vi "_WCA_CLNA_Sweep.vi"(8 "CLNAsweep":T3={"VDmin"=1.0, "VDmax"=2.0, "VDstep"=0.1, "IDmin"=8.0, "IDmax"=20.0, "IDstep"=1.0, "wait (mS)"=500.0, "P.M.aveg"=10, "HOT/COLD "=0, "SIS hotV "=8.0, "SIS coldV"=5.0, "file_name"="", "frq(GHz)"=8.0} {"HOT/COLD" items=["Liq Ni Motor", "SISBias"]}, 10 "Control":T2={"GPIB_ATT"="28", "6501Dev#"=1, "GPIB_SP"="18", "GPIB_PM"="13", "GPIB_DSA"="11", "GPIB_DMM (TPD)"="23", "GPIB_MPI"="2", "mortor設定"=[{"Axis"=0, "ID"=0, "HIspeed"=200.0, "LOspeed"=100.0, "ACCEL(ms)"=100.0, "Sratio"=50.0, "フリーラン\n"=TRUE, "文字列"="DSB HOT/COLD"}, {"Axis"=1, "ID"=0, "HIspeed"=4.0, "LOspeed"=4.0, "ACCEL(ms)"=100.0, "Sratio"=50.0, "フリーラン\n"=TRUE, "文字列"="SubMM Att"}], "DATAパス"=path "Z:/band10/Labview_ALMA/MIX95/test", "DBパス "=path "Z:/band10/Labview_ALMA/MIX95/test", "comment"="P1_Tmin", "ColdCarts"="003601", "Th"=295.0, "Tc"=77.0, "Set_SIS_volt"=2.1, "Offset"=0.0, "control"=0, "FreqLO"=800.0, "Set_Mag_Cur"=800.0, "MPI offset(mm)"=22.99, "HOT/COLD"=0} {"HOT/COLD" items=["DSB", "SBR", "GainComp"]; "control" items=["CLOSE LOOP", "OPEN LOOP", "Not Control"]}, 11 "Bias_LO_equip":T1={"Node address"=19, "CAN Interface"="CAN0", "Cartridge band"=10, "Slave Node in"={"Address"=0, "Serial Number"=[]}, "ObjHandle out"=0, "POL"=1, "sb"=1, "GPIB_SM (SIS S,V)"="24", "GPIB_DMM (SIS I)"="22", "GPIB_SM (MAG I) "="25", "GPIB_SG(LO)"="19", "GPIB_PW (PAMP) "="6", "GPIB_TMP1(8ch)"="12", "GPIB_TMP2(2ch)  "="13", "WCA_avg"=10, "Rsen"=10.0, "BiasModule"=1, "LOModule "=1, "WCA_LO_FREQ_SET"={"YTO Low freq. [GHz]"=14.42, "YTO High freq. [GHz]"=17.7, "Kvco"=1, "Lock Pol."=0, "SET LO FREQ"=72.5, "Multiplier"=6.0, "YTO (HEX)"=0, "YTO coarse( FREQ)"=25.0, "NULL PLL INTEGRATOR"=FALSE}, "Res for"=0} {"Res for" items=["none", "series res", "parallel res"]; "WCA_LO_FREQ_SET"."YTO coarse( FREQ)" min=25 max=150 step=0.0001 format="%.3f"; "WCA_LO_FREQ_SET"."Multiplier" min=3 max=6 step=3; "WCA_LO_FREQ_SET"."SET LO FREQ" min=25 max=150 step=0.0001 format="%.3f"; "WCA_LO_FREQ_SET"."Lock Pol." items=["Lower", "Upper"]; "WCA_LO_FREQ_SET"."Kvco" items=["7.5MHz/V", "15MHz/V"]; "WCA_LO_FREQ_SET"."YTO High freq. [GHz]" format="%.3f"; "WCA_LO_FREQ_SET"."YTO Low freq. [GHz]" format="%.3f"; "LOModule" items=["Manual", "B10Lab LO", "WCA LO"]; "BiasModule" items=["B10Lab Bias", "WCA BiasModule"]; "Slave Node in"."Serial Number" format="%.0x"; "Slave Node in"."Address" format="%.0x"; "Cartridge band" max=10 step=1; "Node address" format="%.0x"}) -> ()   [LabVIEW 2017]
uses:
  __sub_vi/WCA_NAOJ_sub_vi/WCA_Global.vi
  Instance           2 23Saved   _WCA_CLNA_Sweep .vi
  Instance           4 23Saved   _WCA_CLNA_Sweep .vi
  <vilib>/Utility/file.llb/Write To Spreadsheet File (DBL).vi
  <vilib>/express/express shared/transition.llb/Dynamic To Waveform Array.vi
  <vilib>/express/express arith-compare/Formula/Block/exnFormulaBlock how many pts in the wave.vi
  <vilib>/express/express shared/ex_Modify Signal Name.vi
  <vilib>/express/express shared/transition.llb/Waveform Array To Dynamic.vi
  Instance           3 23Saved   _WCA_CLNA_Sweep .vi
  <vilib>/express/express arith-compare/Formula/XNode/ExpressFormulaBlockNode.xnode
panel:
  in  "タブ制御器":enum32{"機器セッティング", "ページ 2", "ページ 3", "ページ 4"}(tab)
  out "Y_":dbl=-0.021313399999996818
  out "Phot":dbl=-36.0813292
  out "Pcold":dbl=-36.0600158
  out "Get VG":dbl=-3.6497344970703125
  out "Get ID":dbl=25.091552734375
  out "Get VD":dbl=2.003662109375
  out "Set ID":dbl=20.0
  out "Set VD":dbl=2.0
  out "error out":errorcluster={"status"=TRUE, "code"=-1074388991, "source"="NI-CAN Wait For State\n(ncWait.vi)"} caption="エラー出力"
  out "Link済み":bool=TRUE
  in  "CLNA_SET":T4 {"SET POL0 LNA1 STAGE3 DRAIN C" min=0 max=20 step=0.01 format="%.2f"; "SET POL0 LNA1 STAGE3 DRAIN V" min=0 max=3 step=0.01 format="%.2f"; "SET POL0 LNA1 STAGE2 DRAIN C" min=0 max=20 step=0.01 format="%.2f"; "SET POL0 LNA1 STAGE2 DRAIN V" min=0 max=3 step=0.01 format="%.2f"; "SET POL0 LNA1 STAGE1 DRAIN C" min=0 max=20 step=0.01 format="%.2f"; "SET POL0 LNA1 STAGE1 DRAIN V" min=0 max=3 step=0.01 format="%.2f"; "CLNA State" items=["Disabled", "Enabled"]}
  out "AllDATA":dbl[][](array[numeric])=[[1.0023040771484375, 1.002105712890625, 1.0022430419921875, 1.0023345947265625, 1.002197265625, 1.0023040771484375, 1.0023956298828125, 1.002227783203125, 1.0021514892578125, 1.0023956298828125, 1.0024871826171875, 1.0022430419921875, 1.0022125244140625, 1.102142333984375, 1.10211181640625, 1.1022491455078125, 1.10211181640625, 1.102294921875, 1.1024169921875, 1.1022796630859375, 1.1022491455078125, 1.1023712158203125, 1.1024017333984375, 1.1024017333984375, 1.1022796630859375, 1.102294921875, 1.2026519775390625, 1.2027435302734375, 1.20269775390625, 1.2028045654296875, 1.2025299072265625, 1.202789306640625, 1.2028656005859375, 1.2028961181640625, 1.2029266357421875, 1.2028656005859375, 1.2026519775390625, 1.2027740478515625, 1.2029266357421875, 1.302642822265625, 1.302703857421875, 1.3027191162109375, 1.302764892578125, 1.3028106689453125, 1.30279541015625, 1.3028106689453125, 1.302978515625, 1.3027496337890625, 1.302825927734375, 1.302642822265625, 1.30291748046875, 1.3028411865234375, 1.4028472900390625, 1.4030914306640625, 1.403167724609375, 1.4028472900390625, 1.4028778076171875, 1.4028778076171875, 1.402679443359375, 1.403076171875, 1.402679443359375, 1.40301513671875, 1.4030914306640625, 1.402984619140625, 1.4026641845703125, 1.503662109375, 1.5032196044921875, 1.50323486328125, 1.5030517578125, 1.5032958984375, 1.5032806396484375, 1.5030364990234375, 1.50335693359375, 1.5030975341796875, 1.5032501220703125, 1.5030517578125, 1.503204345703125, 1.5032196044921875, 1.60296630859375, 1.6030731201171875, 1.603363037109375, 1.6032562255859375, 1.603179931640625, 1.60296630859375, 1.60308837890625, 1.6032562255859375, 1.60308837890625, 1.60321044921875, 1.60321044921875, 1.603057861328125, 1.603118896484375, 1.7034912109375, 1.703216552734375, 1.7032470703125, 1.7033538818359375, 1.7030181884765625, 1.7031097412109375, 1.703460693359375, 1.7033538818359375, 1.70318603515625, 1.7034149169921875, 1.7034759521484375, 1.70306396484375, 1.70343017578125, 1.803375244140625, 1.8035430908203125, 1.8034210205078125, 1.8034515380859375, 1.80340576171875, 1.8035736083984375, 1.8033599853515625, 1.803466796875, 1.8035125732421875, 1.8033599853515625, 1.8035888671875, 1.8033905029296875, 1.8037109375, 1.903350830078125, 1.903472900390625, 1.9034576416015625], [8.008880615234375, 9.035491943359375, 9.97100830078125, 11.0247802734375, 12.0404052734375, 13.050689697265625, 14.05731201171875, 15.0653076171875, 16.02996826171875, 17.058563232421875, 18.0487060546875, 19.04052734375, 20.05828857421875, 8.039398193359375, 8.996124267578125, 10.06439208984375, 11.038818359375, 12.03704833984375, 13.03802490234375, 14.0863037109375, 15.06439208984375, 16.061859130859375, 17.065887451171875, 18.072052001953125, 19.047698974609375, 20.0762939453125, 8.032989501953125, 9.056243896484375, 10.06011962890625, 11.0638427734375, 12.0782470703125, 13.007965087890625, 14.0386962890625, 15.06439208984375, 16.035308837890625, 17.039337158203125, 18.033905029296875, 19.078369140625, 20.070037841796875, 8.048248291015625, 9.024200439453125, 9.9859619140625, 11.053009033203125, 12.051239013671875, 13.049468994140625, 14.071807861328125, 15.03143310546875, 16.085052490234375, 17.037353515625, 18.03558349609375, 19.07135009765625, 20.034027099609375, 7.994232177734375, 9.02862548828125, 10.037841796875, 11.07452392578125, 12.032928466796875, 13.063507080078125, 14.0386962890625, 15.02197265625, 16.014404296875, 17.052001953125, 18.072662353515625, 19.047393798828125, 20.04119873046875, 5.80596923828125, 3.686065673828125, 5.312347412109375, 4.949188232421875, 16.232452392578125, 13.04046630859375, 14.048919677734375, 15.037078857421875, 16.081695556640625, 17.0587158203125, 18.0523681640625, 19.07867431640625, 20.0244140625, 13.279266357421875, 6.36016845703125, 4.31121826171875, 7.32452392578125, 6.24359130859375, 7.073822021484375, 18.690032958984375, 15.014190673828125, 16.087799072265625, 17.076568603515625, 18.069305419921875, 19.0643310546875, 20.07080078125, 8.0560302734375, 8.16162109375, 3.512115478515625, 5.3619384765625, 20.580902099609375, 20.821380615234375, 16.0015869140625, 4.630889892578125, 15.82916259765625, 17.030029296875, 18.027801513671875, 19.0692138671875, 20.095367431640625, 21.844635009765625, 21.697540283203125, 21.622772216796875, 21.66259765625, 21.610870361328125, 21.63330078125, 21.61102294921875, 21.68212890625, 21.672210693359375, 21.784210205078125, 21.6229248046875, 19.026336669921875, 20.05340576171875, 23.668670654296875, 23.538970947265625, 23.544464111328125], [0.7330169677734375, 0.8783721923828125, 1.0079498291015625, 1.1290283203125, 1.2441253662109375, 1.350372314453125, 1.4566192626953125, 1.5489501953125, 1.6483917236328125, 1.746734619140625, 1.853759765625, 1.9870452880859375, 2.1604461669921875, 0.525146484375, 0.680755615234375, 0.8156890869140625, 0.9432830810546875, 1.061859130859375, 1.179656982421875, 1.2897186279296875, 1.4064178466796875, 1.506317138671875, 1.6030120849609375, 1.69744873046875, 1.7970123291015625, 1.901336669921875, 0.2288360595703125, 0.406005859375, 0.5797576904296875, 0.7351226806640625, 0.872039794921875, 0.9920654296875, 1.1099395751953125, 1.22442626953125, 1.33905029296875, 1.4532470703125, 1.55426025390625, 1.6502532958984375, 1.7432403564453125, -0.0763092041015625, 0.1149749755859375, 0.2913055419921875, 0.4664764404296875, 0.630157470703125, 0.7830963134765625, 0.91229248046875, 1.037567138671875, 1.1466217041015625, 1.265960693359375, 1.378326416015625, 1.4917755126953125, 1.594451904296875, -0.3813323974609375, -0.1755523681640625, 0.013671875, 0.186920166015625, 0.349578857421875, 0.50616455078125, 0.6645050048828125, 0.818389892578125, 0.9545440673828125, 1.0711212158203125, 1.1864166259765625, 1.303497314453125, 1.4156951904296875, -1.2528839111328125, -1.786773681640625, -1.2420196533203125, -1.305328369140625, -1.882781982421875, 0.2266998291015625, 0.3792724609375, 0.535247802734375, 0.6952362060546875, 0.84088134765625, 0.9810943603515625, 1.1031036376953125, 1.21795654296875, -2.3688201904296875, -1.410064697265625, -2.0248565673828125, -1.0382232666015625, -1.1384124755859375, -1.006744384765625, -2.1786651611328125, 0.3073883056640625, 0.4534149169921875, 0.5962371826171875, 0.748260498046875, 0.8952178955078125, 1.03143310546875, -1.3086395263671875, -1.2085418701171875, -2.661956787109375, -2.0058746337890625, -2.78607177734375, -3.555145263671875, -1.39764404296875, -1.9747161865234375, -1.3009796142578125, 0.34893798828125, 0.4822540283203125, 0.62396240234375, 0.7726287841796875, -3.6534423828125, -3.6532135009765625, -3.653228759765625, -3.6531982421875, -3.6529541015625, -3.652801513671875, -3.6527252197265625, -3.652679443359375, -3.652496337890625, -3.6523590087890625, -3.652435302734375, 0.3907623291015625, 0.527252197265625, -3.65203857421875, -3.6520233154296875, -3.65191650390625], [-15.8019747, -14.345305, -13.3210423, -12.5917133, -12.0920286, -11.7980894, -11.6930614, -11.7846915, -12.0721581, -12.6224904, -13.7267507, -16.5712959, -21.5777376, -17.0933087, -15.2334231, -13.8489237, -12.8692605, -12.1592133, -11.639288, -11.2830662, -11.0867126, -11.0497694, -11.1765261, -11.5024369, -12.0712356, -13.1210202, -18.6468403, -16.1476854, -14.570121, -13.4081903, -12.4958806, -11.8057103, -11.2893617, -10.90672, -10.6370429, -10.4946825, -10.494992, -10.6523369, -10.9887522, -22.5221729, -18.125333, -15.4214337, -13.9034386, -12.8769868, -12.1038889, -11.4548295, -10.9493002, -10.5603601, -10.272209, -10.0697857, -9.98018936, -10.0091371, -27.7214104, -22.9626936, -18.0779783, -15.2169109, -13.537981, -12.4632357, -11.7336743, -11.1640832, -10.6783089, -10.3048974, -10.0043142, -9.78552749, -9.63525648, -29.9236072, -30.0847895, -30.3171631, -30.3069408, -30.5019806, -13.4081314, -12.1836691, -11.3858437, -10.8426287, -10.4020521, -10.0248496, -9.71805946, -9.50416462, -28.864449, -30.5298938, -29.3480611, -30.7227796, -30.9749093, -30.1810534, -30.4759237, -11.8363611, -11.0494144, -10.4770986, -10.0581157, -9.73425389, -9.45626546, -28.7626425, -29.4905465, -28.7472986, -30.4154173, -29.8859621, -31.9666589, -30.5494954, -30.5235955, -31.7679326, -10.9375712, -10.3127095, -9.84276742, -9.48202177, -34.5858391, -34.5288413, -34.3235417, -34.3295835, -34.5159358, -34.3741306, -34.4705043, -34.5540513, -34.4242323, -34.5184065, -27.8331629, -10.1602425, -9.68344682, -35.2753216, -35.3063507, -35.2783414], [-18.1174805, -16.6835391, -15.6987861, -14.9944898, -14.5063113, -14.2123343, -14.104885, -14.1915152, -14.4719556, -15.0076862, -16.0726006, -18.7799405, -23.2595732, -19.2586723, -17.5333956, -16.2048421, -15.2456024, -14.556834, -14.049878, -13.692676, -13.4852123, -13.4535138, -13.5758048, -13.8915443, -14.4403795, -15.4600873, -20.6351209, -18.3316269, -16.8141631, -15.7405915, -14.8552992, -14.1820555, -13.6803907, -13.296921, -13.0340352, -12.8908561, -12.8921382, -13.0431259, -13.3727695, -23.9303013, -20.0681201, -17.6391096, -16.1885809, -15.2049061, -14.4666364, -13.8254901, -13.3183269, -12.9474389, -12.6593856, -12.4648366, -12.3737855, -12.6038004, -27.8709028, -24.0548698, -19.9170932, -17.3075996, -15.8115317, -14.7876725, -14.079908, -13.527917, -13.0683468, -12.6767887, -12.3950819, -12.1703213, -12.0184709, -29.8978082, -29.5950189, -30.1216617, -30.2923534, -30.7282828, -15.6183781, -14.4711486, -13.7208693, -13.1918311, -12.762488, -12.4131872, -12.1016409, -11.8839305, -28.9212261, -29.0167155, -29.6828341, -31.0176264, -30.2920578, -30.9538346, -30.4441937, -14.1155557, -13.3635281, -12.8309223, -12.4244692, -12.1112123, -11.8309856, -28.8106043, -30.8510766, -29.2806575, -31.1178272, -31.2416511, -29.5672254, -29.902671, -30.8986962, -31.7747404, -13.220053, -12.6236218, -12.1768264, -11.8501035, -34.4679122, -34.4354168, -28.5827453, -34.491634, -34.4472451, -34.5085919, -34.4868301, -34.2848253, -34.4136795, -34.4331047, -13.1088166, -12.4595201, -12.0024162, -35.4359339, -35.4317712, -35.3773834], [2.3155057999999986, 2.338234100000001, 2.3777437999999993, 2.4027765, 2.4142826999999993, 2.4142449, 2.4118236, 2.4068237000000003, 2.3997975, 2.3851958, 2.345849900000001, 2.2086445999999995, 1.6818355999999994, 2.165363599999999, 2.299972499999999, 2.3559184, 2.3763419, 2.397620700000001, 2.410589999999999, 2.4096098, 2.3984997000000003, 2.403744399999999, 2.3992787, 2.3891074000000003, 2.369143900000001, 2.3390670999999994, 1.9882805999999995, 2.1839414999999995, 2.244042099999998, 2.3324012000000014, 2.3594185999999997, 2.376345200000001, 2.3910289999999996, 2.3902009999999994, 2.396992299999999, 2.396173600000001, 2.3971462, 2.390789, 2.3840173, 1.408128399999999, 1.9427871000000003, 2.2176759000000015, 2.285142300000002, 2.3279193000000014, 2.362747500000001, 2.370660599999999, 2.369026700000001, 2.3870787999999994, 2.3871766, 2.3950508999999993, 2.3935961399999997, 2.5946633000000006, 0.14949239999999975, 1.0921761999999973, 1.8391148999999984, 2.0906886999999994, 2.2735506999999995, 2.324436799999999, 2.346233699999999, 2.3638338, 2.390037900000001, 2.3718912999999997, 2.3907676999999996, 2.3847938099999997, 2.38321442, -0.02579899999999924, -0.48977059999999994, -0.19550139999999772, -0.014587399999999917, 0.22630219999999923, 2.210246699999999, 2.2874795, 2.3350256, 2.3492023999999994, 2.360435899999999, 2.3883376, 2.3835814400000004, 2.3797658800000008, 0.056777099999997915, -1.5131782999999999, 0.334773000000002, 0.29484680000000196, -0.6828515000000017, 0.7727812000000007, -0.03172999999999959, 2.2791946000000003, 2.3141137, 2.3538236999999995, 2.3663535000000007, 2.3769584100000003, 2.374720140000001, 0.04796180000000305, 1.3605300999999983, 0.5333588999999996, 0.7024098999999993, 1.3556889999999981, -2.399433499999997, -0.6468243999999999, 0.37510070000000084, 0.006807799999997144, 2.2824817999999993, 2.3109123, 2.33405898, 2.36808173, -0.1179269000000005, -0.09342450000000468, -5.740796400000001, 0.16205049999999943, -0.06869069999999766, 0.13446129999999812, 0.01632579999999706, -0.2692259999999962, -0.010552799999999252, -0.08530179999999632, -14.7243463, 2.2992776, 2.3189693800000004, 0.16061230000000393, 0.12542049999999705, 0.09904199999999719]]
  out "GETID2d":dbl[][](array[numeric])=[[8.008880615234375, 9.035491943359375, 9.97100830078125, 11.0247802734375, 12.0404052734375, 13.050689697265625, 14.05731201171875, 15.0653076171875, 16.02996826171875, 17.058563232421875, 18.0487060546875, 19.04052734375, 20.05828857421875], [8.039398193359375, 8.996124267578125, 10.06439208984375, 11.038818359375, 12.03704833984375, 13.03802490234375, 14.0863037109375, 15.06439208984375, 16.061859130859375, 17.065887451171875, 18.072052001953125, 19.047698974609375, 20.0762939453125], [8.032989501953125, 9.056243896484375, 10.06011962890625, 11.0638427734375, 12.0782470703125, 13.007965087890625, 14.0386962890625, 15.06439208984375, 16.035308837890625, 17.039337158203125, 18.033905029296875, 19.078369140625, 20.070037841796875], [8.048248291015625, 9.024200439453125, 9.9859619140625, 11.053009033203125, 12.051239013671875, 13.049468994140625, 14.071807861328125, 15.03143310546875, 16.085052490234375, 17.037353515625, 18.03558349609375, 19.07135009765625, 20.034027099609375], [7.994232177734375, 9.02862548828125, 10.037841796875, 11.07452392578125, 12.032928466796875, 13.063507080078125, 14.0386962890625, 15.02197265625, 16.014404296875, 17.052001953125, 18.072662353515625, 19.047393798828125, 20.04119873046875], [5.80596923828125, 3.686065673828125, 5.312347412109375, 4.949188232421875, 16.232452392578125, 13.04046630859375, 14.048919677734375, 15.037078857421875, 16.081695556640625, 17.0587158203125, 18.0523681640625, 19.07867431640625, 20.0244140625], [13.279266357421875, 6.36016845703125, 4.31121826171875, 7.32452392578125, 6.24359130859375, 7.073822021484375, 18.690032958984375, 15.014190673828125, 16.087799072265625, 17.076568603515625, 18.069305419921875, 19.0643310546875, 20.07080078125], [8.0560302734375, 8.16162109375, 3.512115478515625, 5.3619384765625, 20.580902099609375, 20.821380615234375, 16.0015869140625, 4.630889892578125, 15.82916259765625, 17.030029296875, 18.027801513671875, 19.0692138671875, 20.095367431640625], [21.844635009765625, 21.697540283203125, 21.622772216796875, 21.66259765625, 21.610870361328125, 21.63330078125, 21.61102294921875, 21.68212890625, 21.672210693359375, 21.784210205078125, 21.6229248046875, 19.026336669921875, 20.05340576171875], [23.668670654296875, 23.538970947265625, 23.544464111328125, 23.495635986328125, 23.45367431640625, 23.48358154296875, 23.45367431640625, 23.459625244140625, 23.370819091796875, 23.431549072265625, 23.40972900390625, 23.4197998046875, 23.384552001953125], [25.102386474609375, 25.07843017578125, 25.081787109375, 25.060577392578125, 25.09002685546875, 25.065460205078125, 25.092620849609375, 25.110015869140625, 25.070648193359375, 25.105438232421875, 25.09002685546875, 25.069732666015625, 25.091552734375]]
  out "GetVD 2D":dbl[][](array[numeric])=[[1.0023040771484375, 1.002105712890625, 1.0022430419921875, 1.0023345947265625, 1.002197265625, 1.0023040771484375, 1.0023956298828125, 1.002227783203125, 1.0021514892578125, 1.0023956298828125, 1.0024871826171875, 1.0022430419921875, 1.0022125244140625], [1.102142333984375, 1.10211181640625, 1.1022491455078125, 1.10211181640625, 1.102294921875, 1.1024169921875, 1.1022796630859375, 1.1022491455078125, 1.1023712158203125, 1.1024017333984375, 1.1024017333984375, 1.1022796630859375, 1.102294921875], [1.2026519775390625, 1.2027435302734375, 1.20269775390625, 1.2028045654296875, 1.2025299072265625, 1.202789306640625, 1.2028656005859375, 1.2028961181640625, 1.2029266357421875, 1.2028656005859375, 1.2026519775390625, 1.2027740478515625, 1.2029266357421875], [1.302642822265625, 1.302703857421875, 1.3027191162109375, 1.302764892578125, 1.3028106689453125, 1.30279541015625, 1.3028106689453125, 1.302978515625, 1.3027496337890625, 1.302825927734375, 1.302642822265625, 1.30291748046875, 1.3028411865234375], [1.4028472900390625, 1.4030914306640625, 1.403167724609375, 1.4028472900390625, 1.4028778076171875, 1.4028778076171875, 1.402679443359375, 1.403076171875, 1.402679443359375, 1.40301513671875, 1.4030914306640625, 1.402984619140625, 1.4026641845703125], [1.503662109375, 1.5032196044921875, 1.50323486328125, 1.5030517578125, 1.5032958984375, 1.5032806396484375, 1.5030364990234375, 1.50335693359375, 1.5030975341796875, 1.5032501220703125, 1.5030517578125, 1.503204345703125, 1.5032196044921875], [1.60296630859375, 1.6030731201171875, 1.603363037109375, 1.6032562255859375, 1.603179931640625, 1.60296630859375, 1.60308837890625, 1.6032562255859375, 1.60308837890625, 1.60321044921875, 1.60321044921875, 1.603057861328125, 1.603118896484375], [1.7034912109375, 1.703216552734375, 1.7032470703125, 1.7033538818359375, 1.7030181884765625, 1.7031097412109375, 1.703460693359375, 1.7033538818359375, 1.70318603515625, 1.7034149169921875, 1.7034759521484375, 1.70306396484375, 1.70343017578125], [1.803375244140625, 1.8035430908203125, 1.8034210205078125, 1.8034515380859375, 1.80340576171875, 1.8035736083984375, 1.8033599853515625, 1.803466796875, 1.8035125732421875, 1.8033599853515625, 1.8035888671875, 1.8033905029296875, 1.8037109375], [1.903350830078125, 1.903472900390625, 1.9034576416015625, 1.9034271240234375, 1.903411865234375, 1.9035491943359375, 1.903472900390625, 1.9034881591796875, 1.9035186767578125, 1.903564453125, 1.9035797119140625, 1.9035491943359375, 1.903717041015625], [2.0036773681640625, 2.0038909912109375, 2.003662109375, 2.0037078857421875, 2.003814697265625, 2.0035552978515625, 2.0036163330078125, 2.0038909912109375, 2.003753662109375, 2.0037994384765625, 2.003692626953125, 2.0037689208984375, 2.003662109375]]
  out "Y":dbl[][](array[numeric])=[[2.3155057999999986, 2.338234100000001, 2.3777437999999993, 2.4027765, 2.4142826999999993, 2.4142449, 2.4118236, 2.4068237000000003, 2.3997975, 2.3851958, 2.345849900000001, 2.2086445999999995, 1.6818355999999994], [2.165363599999999, 2.299972499999999, 2.3559184, 2.3763419, 2.397620700000001, 2.410589999999999, 2.4096098, 2.3984997000000003, 2.403744399999999, 2.3992787, 2.3891074000000003, 2.369143900000001, 2.3390670999999994], [1.9882805999999995, 2.1839414999999995, 2.244042099999998, 2.3324012000000014, 2.3594185999999997, 2.376345200000001, 2.3910289999999996, 2.3902009999999994, 2.396992299999999, 2.396173600000001, 2.3971462, 2.390789, 2.3840173], [1.408128399999999, 1.9427871000000003, 2.2176759000000015, 2.285142300000002, 2.3279193000000014, 2.362747500000001, 2.370660599999999, 2.369026700000001, 2.3870787999999994, 2.3871766, 2.3950508999999993, 2.3935961399999997, 2.5946633000000006], [0.14949239999999975, 1.0921761999999973, 1.8391148999999984, 2.0906886999999994, 2.2735506999999995, 2.324436799999999, 2.346233699999999, 2.3638338, 2.390037900000001, 2.3718912999999997, 2.3907676999999996, 2.3847938099999997, 2.38321442], [-0.02579899999999924, -0.48977059999999994, -0.19550139999999772, -0.014587399999999917, 0.22630219999999923, 2.210246699999999, 2.2874795, 2.3350256, 2.3492023999999994, 2.360435899999999, 2.3883376, 2.3835814400000004, 2.3797658800000008], [0.056777099999997915, -1.5131782999999999, 0.334773000000002, 0.29484680000000196, -0.6828515000000017, 0.7727812000000007, -0.03172999999999959, 2.2791946000000003, 2.3141137, 2.3538236999999995, 2.3663535000000007, 2.3769584100000003, 2.374720140000001], [0.04796180000000305, 1.3605300999999983, 0.5333588999999996, 0.7024098999999993, 1.3556889999999981, -2.399433499999997, -0.6468243999999999, 0.37510070000000084, 0.006807799999997144, 2.2824817999999993, 2.3109123, 2.33405898, 2.36808173], [-0.1179269000000005, -0.09342450000000468, -5.740796400000001, 0.16205049999999943, -0.06869069999999766, 0.13446129999999812, 0.01632579999999706, -0.2692259999999962, -0.010552799999999252, -0.08530179999999632, -14.7243463, 2.2992776, 2.3189693800000004], [0.16061230000000393, 0.12542049999999705, 0.09904199999999719, -0.09832660000000004, 0.06042730000000063, -0.013606299999999294, 0.09472170000000091, -0.01313999999999993, 0.03965420000000108, -0.0711752000000061, -0.057129299999999716, -0.187052400000006, 0.24542750000000524], [0.10479219999999856, -0.022885199999997496, 0.19579489999999566, -0.05049950000000081, -0.08708850000000012, -0.0541388999999981, -0.1317682999999974, 0.21901909999999702, 0.07415780000000183, -0.03721460000000576, -0.29298759999999646, 0.13120839999999845, -0.021313399999996818]]
  out "PC":dbl[][](array[numeric])=[[-18.1174805, -16.6835391, -15.6987861, -14.9944898, -14.5063113, -14.2123343, -14.104885, -14.1915152, -14.4719556, -15.0076862, -16.0726006, -18.7799405, -23.2595732], [-19.2586723, -17.5333956, -16.2048421, -15.2456024, -14.556834, -14.049878, -13.692676, -13.4852123, -13.4535138, -13.5758048, -13.8915443, -14.4403795, -15.4600873], [-20.6351209, -18.3316269, -16.8141631, -15.7405915, -14.8552992, -14.1820555, -13.6803907, -13.296921, -13.0340352, -12.8908561, -12.8921382, -13.0431259, -13.3727695], [-23.9303013, -20.0681201, -17.6391096, -16.1885809, -15.2049061, -14.4666364, -13.8254901, -13.3183269, -12.9474389, -12.6593856, -12.4648366, -12.3737855, -12.6038004], [-27.8709028, -24.0548698, -19.9170932, -17.3075996, -15.8115317, -14.7876725, -14.079908, -13.527917, -13.0683468, -12.6767887, -12.3950819, -12.1703213, -12.0184709], [-29.8978082, -29.5950189, -30.1216617, -30.2923534, -30.7282828, -15.6183781, -14.4711486, -13.7208693, -13.1918311, -12.762488, -12.4131872, -12.1016409, -11.8839305], [-28.9212261, -29.0167155, -29.6828341, -31.0176264, -30.2920578, -30.9538346, -30.4441937, -14.1155557, -13.3635281, -12.8309223, -12.4244692, -12.1112123, -11.8309856], [-28.8106043, -30.8510766, -29.2806575, -31.1178272, -31.2416511, -29.5672254, -29.902671, -30.8986962, -31.7747404, -13.220053, -12.6236218, -12.1768264, -11.8501035], [-34.4679122, -34.4354168, -28.5827453, -34.491634, -34.4472451, -34.5085919, -34.4868301, -34.2848253, -34.4136795, -34.4331047, -13.1088166, -12.4595201, -12.0024162], [-35.4359339, -35.4317712, -35.3773834, -35.244766, -35.411508, -35.3262657, -35.3884755, -35.31755, -35.3399327, -35.3057726, -35.3903215, -35.203278, -35.4838991], [-36.0377979, -36.1185581, -36.1441532, -35.9787072, -35.9739156, -35.9864678, -36.0065619, -36.1079155, -36.091712, -35.9935401, -35.892561, -36.105768, -36.0600158]]
  out "PH":dbl[][](array[numeric])=[[-15.8019747, -14.345305, -13.3210423, -12.5917133, -12.0920286, -11.7980894, -11.6930614, -11.7846915, -12.0721581, -12.6224904, -13.7267507, -16.5712959, -21.5777376], [-17.0933087, -15.2334231, -13.8489237, -12.8692605, -12.1592133, -11.639288, -11.2830662, -11.0867126, -11.0497694, -11.1765261, -11.5024369, -12.0712356, -13.1210202], [-18.6468403, -16.1476854, -14.570121, -13.4081903, -12.4958806, -11.8057103, -11.2893617, -10.90672, -10.6370429, -10.4946825, -10.494992, -10.6523369, -10.9887522], [-22.5221729, -18.125333, -15.4214337, -13.9034386, -12.8769868, -12.1038889, -11.4548295, -10.9493002, -10.5603601, -10.272209, -10.0697857, -9.98018936, -10.0091371], [-27.7214104, -22.9626936, -18.0779783, -15.2169109, -13.537981, -12.4632357, -11.7336743, -11.1640832, -10.6783089, -10.3048974, -10.0043142, -9.78552749, -9.63525648], [-29.9236072, -30.0847895, -30.3171631, -30.3069408, -30.5019806, -13.4081314, -12.1836691, -11.3858437, -10.8426287, -10.4020521, -10.0248496, -9.71805946, -9.50416462], [-28.864449, -30.5298938, -29.3480611, -30.7227796, -30.9749093, -30.1810534, -30.4759237, -11.8363611, -11.0494144, -10.4770986, -10.0581157, -9.73425389, -9.45626546], [-28.7626425, -29.4905465, -28.7472986, -30.4154173, -29.8859621, -31.9666589, -30.5494954, -30.5235955, -31.7679326, -10.9375712, -10.3127095, -9.84276742, -9.48202177], [-34.5858391, -34.5288413, -34.3235417, -34.3295835, -34.5159358, -34.3741306, -34.4705043, -34.5540513, -34.4242323, -34.5184065, -27.8331629, -10.1602425, -9.68344682], [-35.2753216, -35.3063507, -35.2783414, -35.3430926, -35.3510807, -35.339872, -35.2937538, -35.33069, -35.3002785, -35.3769478, -35.4474508, -35.3903304, -35.2384716], [-35.9330057, -36.1414433, -35.9483583, -36.0292067, -36.0610041, -36.0406067, -36.1383302, -35.8888964, -36.0175542, -36.0307547, -36.1855486, -35.9745596, -36.0813292]]
  out "VG":dbl[][](array[numeric])=[[0.7330169677734375, 0.8783721923828125, 1.0079498291015625, 1.1290283203125, 1.2441253662109375, 1.350372314453125, 1.4566192626953125, 1.5489501953125, 1.6483917236328125, 1.746734619140625, 1.853759765625, 1.9870452880859375, 2.1604461669921875], [0.525146484375, 0.680755615234375, 0.8156890869140625, 0.9432830810546875, 1.061859130859375, 1.179656982421875, 1.2897186279296875, 1.4064178466796875, 1.506317138671875, 1.6030120849609375, 1.69744873046875, 1.7970123291015625, 1.901336669921875], [0.2288360595703125, 0.406005859375, 0.5797576904296875, 0.7351226806640625, 0.872039794921875, 0.9920654296875, 1.1099395751953125, 1.22442626953125, 1.33905029296875, 1.4532470703125, 1.55426025390625, 1.6502532958984375, 1.7432403564453125], [-0.0763092041015625, 0.1149749755859375, 0.2913055419921875, 0.4664764404296875, 0.630157470703125, 0.7830963134765625, 0.91229248046875, 1.037567138671875, 1.1466217041015625, 1.265960693359375, 1.378326416015625, 1.4917755126953125, 1.594451904296875], [-0.3813323974609375, -0.1755523681640625, 0.013671875, 0.186920166015625, 0.349578857421875, 0.50616455078125, 0.6645050048828125, 0.818389892578125, 0.9545440673828125, 1.0711212158203125, 1.1864166259765625, 1.303497314453125, 1.4156951904296875], [-1.2528839111328125, -1.786773681640625, -1.2420196533203125, -1.305328369140625, -1.882781982421875, 0.2266998291015625, 0.3792724609375, 0.535247802734375, 0.6952362060546875, 0.84088134765625, 0.9810943603515625, 1.1031036376953125, 1.21795654296875], [-2.3688201904296875, -1.410064697265625, -2.0248565673828125, -1.0382232666015625, -1.1384124755859375, -1.006744384765625, -2.1786651611328125, 0.3073883056640625, 0.4534149169921875, 0.5962371826171875, 0.748260498046875, 0.8952178955078125, 1.03143310546875], [-1.3086395263671875, -1.2085418701171875, -2.661956787109375, -2.0058746337890625, -2.78607177734375, -3.555145263671875, -1.39764404296875, -1.9747161865234375, -1.3009796142578125, 0.34893798828125, 0.4822540283203125, 0.62396240234375, 0.7726287841796875], [-3.6534423828125, -3.6532135009765625, -3.653228759765625, -3.6531982421875, -3.6529541015625, -3.652801513671875, -3.6527252197265625, -3.652679443359375, -3.652496337890625, -3.6523590087890625, -3.652435302734375, 0.3907623291015625, 0.527252197265625], [-3.65203857421875, -3.6520233154296875, -3.65191650390625, -3.6517791748046875, -3.651824951171875, -3.651702880859375, -3.65155029296875, -3.65155029296875, -3.6516265869140625, -3.6514434814453125, -3.65142822265625, -3.6511688232421875, -3.6511993408203125], [-3.6509552001953125, -3.6507415771484375, -3.6507110595703125, -3.650726318359375, -3.6506500244140625, -3.6505279541015625, -3.6504364013671875, -3.6502532958984375, -3.6502685546875, -3.650115966796875, -3.6500396728515625, -3.650054931640625, -3.6497344970703125]]
  out "SET VD":dbl[](array[numeric])=[1.0, 1.1, 1.2, 1.3, 1.4, 1.5, 1.6, 1.7000000000000002, 1.8, 1.9, 2.0]
  out "SET ID":dbl[](array[numeric])=[8.0, 9.0, 10.0, 11.0, 12.0, 13.0, 14.0, 15.0, 16.0, 17.0, 18.0, 19.0, 20.0]
  # "LO freq. [GHz]"
  # "YTO LOW\n/High Freq."
  # "ZERO Intgrtr"
  # "Node Address"
  # "Serial Number"
  # "Vd [V]"
  # "Id [mA]"
  # "Stage 1"
  # "Stage 2"
  # "Stage 3"
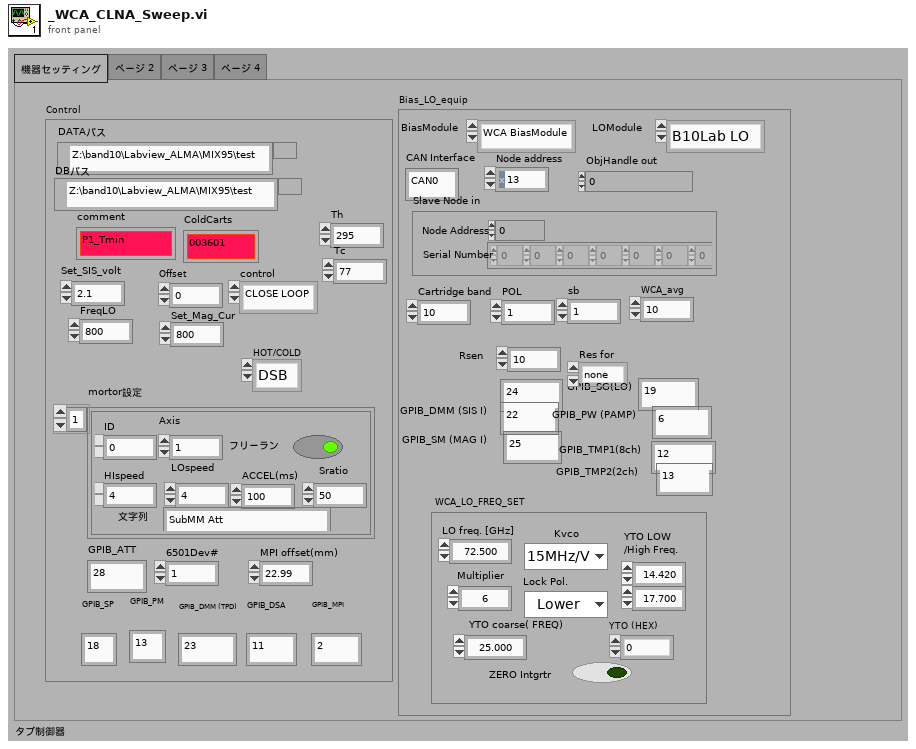
[diagram p1: front panel]
types:
  T1 = cluster{"Node address":u16, "CAN Interface":string, "Cartridge band":u32, "Slave Node in":cluster{"Address":i16, "Serial Number":i8[]}, "ObjHandle out":u32, "POL":u32, "sb":u32, "GPIB_SM (SIS S,V)":string, "GPIB_DMM (SIS I)":string, "GPIB_SM (MAG I) ":string, "GPIB_SG(LO)":string, "GPIB_PW (PAMP) ":string, "GPIB_TMP1(8ch)":string, "GPIB_TMP2(2ch)  ":string, "WCA_avg":i32, "Rsen":dbl, "BiasModule":u16, "LOModule ":u16, "WCA_LO_FREQ_SET":cluster{"YTO Low freq. [GHz]":sgl, "YTO High freq. [GHz]":sgl, "Kvco":u16, "Lock Pol.":u16, "SET LO FREQ":sgl, "Multiplier":sgl, "YTO (HEX)":u16, "YTO coarse( FREQ)":sgl, "NULL PLL INTEGRATOR":bool}, "Res for":u16}
  T2 = cluster{"GPIB_ATT":string, "6501Dev#":i16, "GPIB_SP":string, "GPIB_PM":string, "GPIB_DSA":string, "GPIB_DMM (TPD)":string, "GPIB_MPI":string, "mortor設定":cluster{"Axis":i16, "ID":i16, "HIspeed":dbl, "LOspeed":dbl, "ACCEL(ms)":dbl, "Sratio":dbl, "フリーラン\n":bool, "文字列":string}[], "DATAパス":path, "DBパス ":path, "comment":string, "ColdCarts":string, "Th":dbl, "Tc":dbl, "Set_SIS_volt":dbl, "Offset":dbl, "control":u16, "FreqLO":dbl, "Set_Mag_Cur":dbl, "MPI offset(mm)":dbl, "HOT/COLD":u16}
  T3 = cluster{"VDmin":dbl, "VDmax":dbl, "VDstep":dbl, "IDmin":dbl, "IDmax":dbl, "IDstep":dbl, "wait (mS)":dbl, "P.M.aveg":i32, "HOT/COLD ":u16, "SIS hotV ":dbl, "SIS coldV":dbl, "file_name":string, "frq(GHz)":dbl}
  T4 = cluster{"CLNA State":u8, "SET POL0 LNA1 STAGE1 DRAIN V":sgl, "SET POL0 LNA1 STAGE1 DRAIN C":sgl, "SET POL0 LNA1 STAGE2 DRAIN V":sgl, "SET POL0 LNA1 STAGE2 DRAIN C":sgl, "SET POL0 LNA1 STAGE3 DRAIN V":sgl, "SET POL0 LNA1 STAGE3 DRAIN C":sgl}
  T5 = cluster{"Axis":i16, "ID":i16, "HIspeed":dbl, "LOspeed":dbl, "ACCEL(ms)":dbl, "Sratio":dbl, "フリーラン\n":bool, "文字列":string}[]
  T6 = cluster{"Axis":i16, "ID":i16, "HIspeed":dbl, "LOspeed":dbl, "ACCEL(ms)":dbl, "Sratio":dbl, "フリーラン\n":bool, "文字列":string}
  T7 = cluster{"Pol0 LNA1 S1 Drain V [V]":sgl, "Pol0 LNA1 S1 Drain C [mA]":sgl, "Pol0 LNA1 S1 Gate V [V]":sgl, "Pol0 LNA1 S2 Drain V [V]":sgl, "Pol0 LNA1 S2 Drain C [mA]":sgl, "Pol0 LNA1 S2 Gate V [V]":sgl, "Pol0 LNA1 S3 Drain V [V]":sgl, "Pol0 LNA1 S3 Drain C [mA]":sgl, "Pol0 LNA1 S3 Gate V [V]":sgl, "Pol0 LNA1 State":enum16{"Disabled", "Enabled"}}
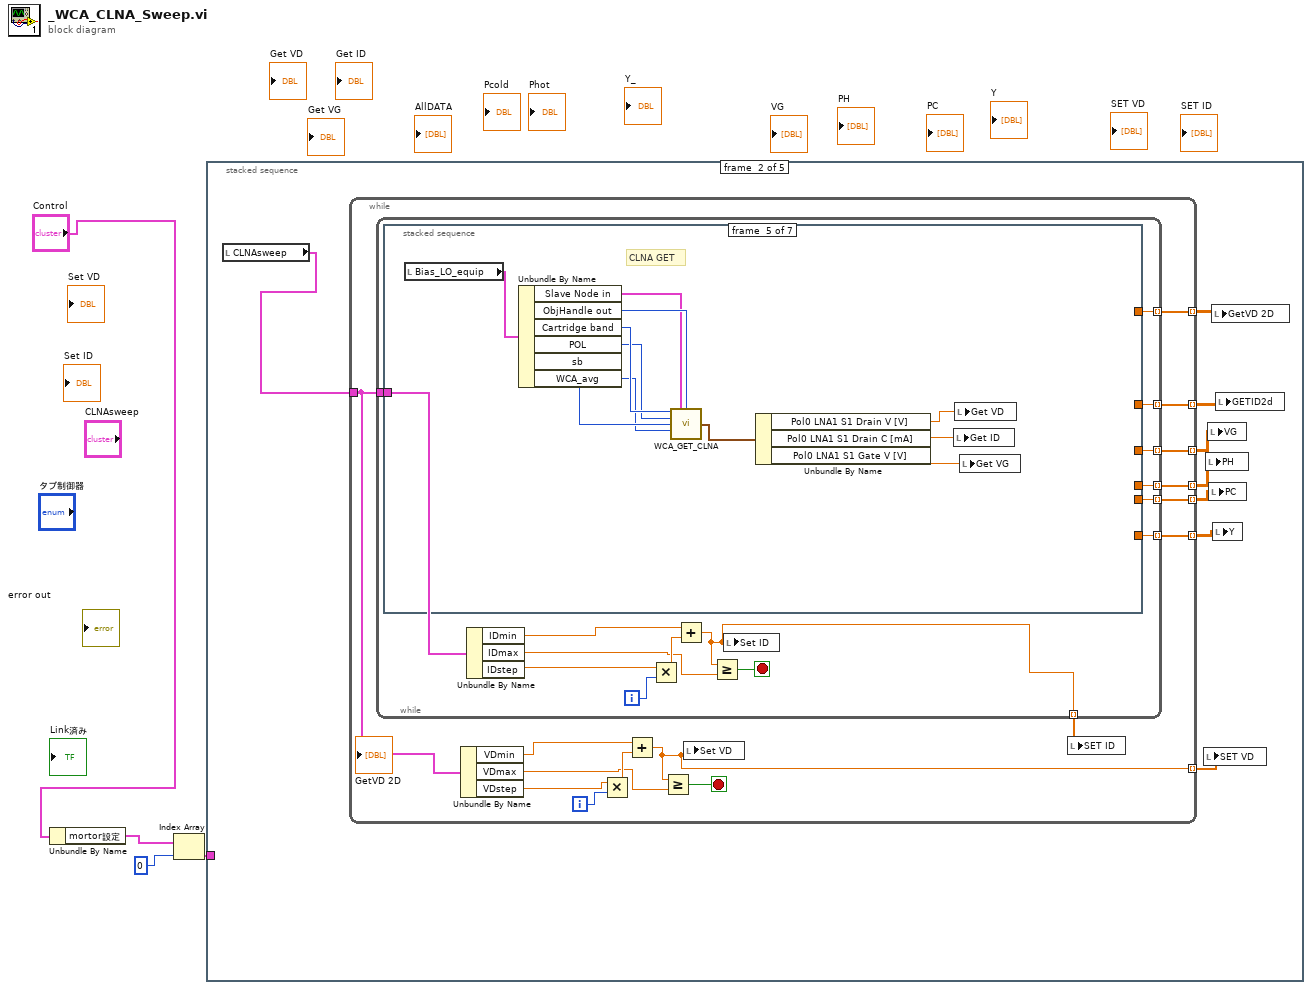
[diagram p0: block diagram]
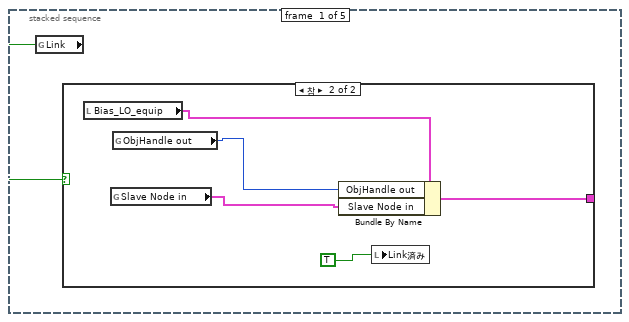
[diagram p2: hidden frame]
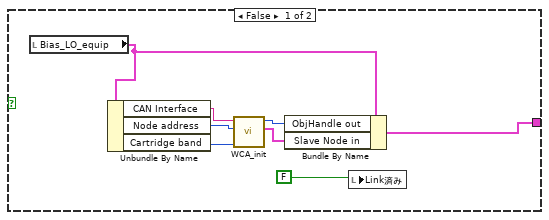
[diagram p3: hidden frame]
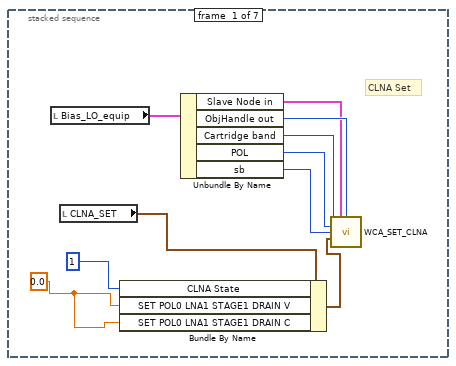
[diagram p4: hidden frame]
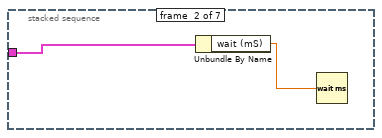
[diagram p5: hidden frame]
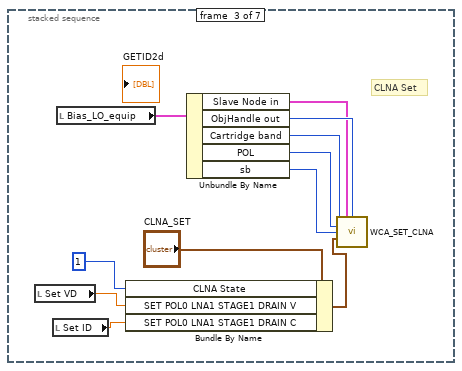
[diagram p6: hidden frame]
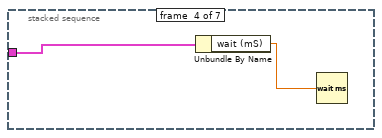
[diagram p7: hidden frame]
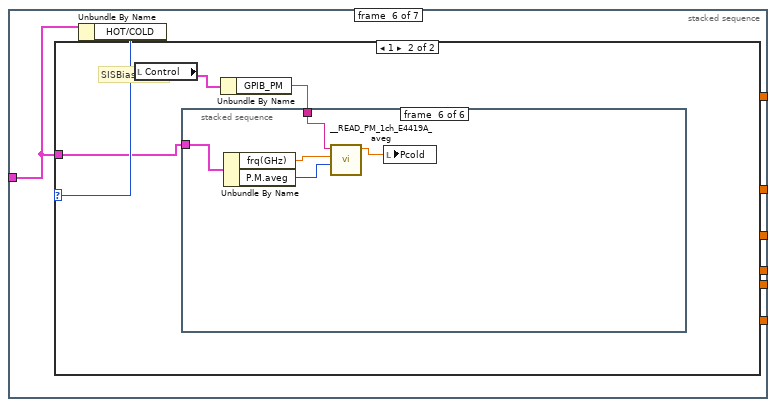
[diagram p8: hidden frame]
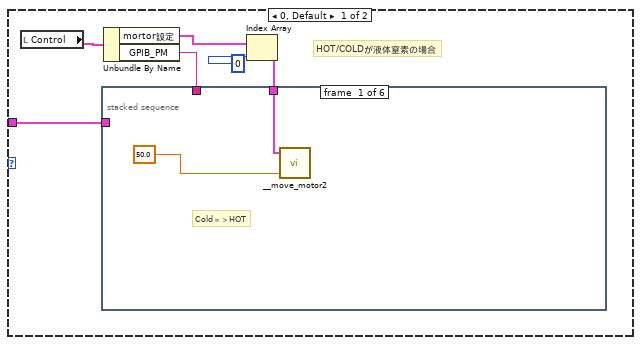
[diagram p9: hidden frame]
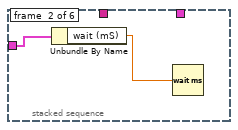
[diagram p10: hidden frame]
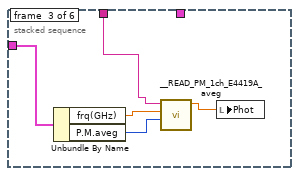
[diagram p11: hidden frame]
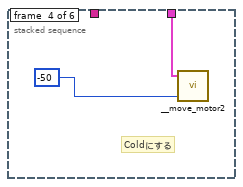
[diagram p12: hidden frame]
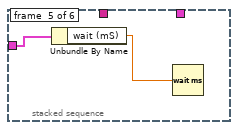
[diagram p13: hidden frame]
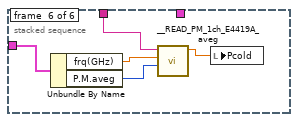
[diagram p14: hidden frame]
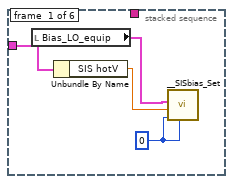
[diagram p15: hidden frame]
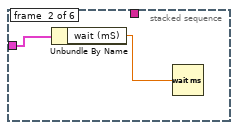
[diagram p16: hidden frame]
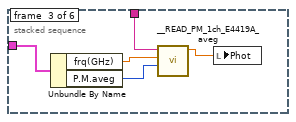
[diagram p17: hidden frame]
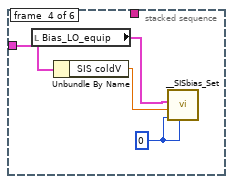
[diagram p18: hidden frame]
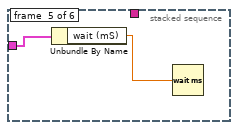
[diagram p19: hidden frame]
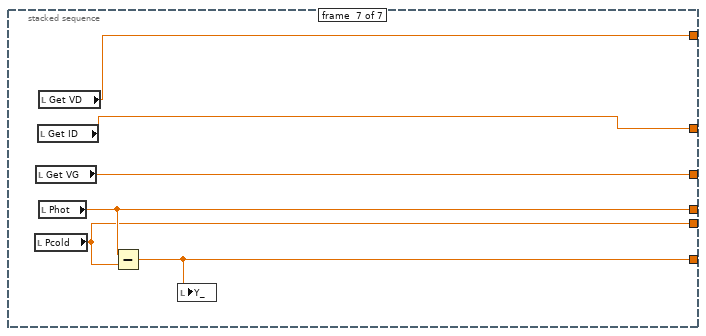
[diagram p20: hidden frame]
diagram:
  n1 = Unbundle By Name("Control") -> ("mortor設定"=w4:T5)
  n2 = Index Array(array=w4, index=0) -> (element=w2:T6)
  n3 = stacked-sequence {
    tunnel: w2 -> [_ _ _ _ _]
    frame #0 {
      n4 = global read "WCA_Global.vi" "Link"() -> (w5:bool)
      n5 = case shown="참" w5 {
        tunnel: [w6 w14] -> _
        frame False {
          n6 = local read "Bias_LO_equip"() -> (w8:T1)
          n7 = Unbundle By Name(w8) -> ("CAN Interface"=w11:string, "Node address"=w10:u16, "Cartridge band"=w9:u32)
          n8 = call "WCA_init.vi"("Cartridge band"=w9, "Node address"=w10, "CAN Interface"=w11) -> ("Slave Node in"=w12:cluster{"Address":i16, "Serial Number":i8[]}, "ObjHandle out"=w13:u32)  [unwired: 4 in, 3 out]
          n9 = Bundle By Name(cluster=w8, "ObjHandle out"=w13, "Slave Node in"=w12) -> (w6:T1)
          n10 = local write "Link済み"(FALSE) -> ()
        }
        frame True {
          n11 = local read "Bias_LO_equip"() -> (w18:T1)
          n12 = global read "WCA_Global.vi" "Slave Node in"() -> (w16:cluster{"Address":i16, "Serial Number":i8[]})
          n13 = global read "WCA_Global.vi" "ObjHandle out"() -> (w17:u32)
          n14 = Bundle By Name(cluster=w18, "ObjHandle out"=w17, "Slave Node in"=w16) -> (w14:T1)
          n15 = local write "Link済み"(TRUE) -> ()
        }
      }
    }
    frame #1 {
      n16 = local read "CLNAsweep"() -> (w26:T3)
      n17 = while {
        tunnel: w26 -> [w35]
        tunnel: [w34] -> w20 mode=indexing
        tunnel: [w33] -> w19 mode=indexing
        tunnel: [w32] -> w25 mode=indexing
        tunnel: [w31] -> w24 mode=indexing
        tunnel: [w30] -> w23 mode=indexing
        tunnel: [w29] -> w22 mode=indexing
        tunnel: [w27] -> w21 mode=indexing
        i -> [w41]
        stop <- w39 stop-if-true
        n18 = while {
          tunnel: w35 -> [w49]
          tunnel: [w48] -> w34 mode=indexing
          tunnel: [w47] -> w33 mode=indexing
          tunnel: [w46] -> w32 mode=indexing
          tunnel: [w45] -> w31 mode=indexing
          tunnel: [w44] -> w30 mode=indexing
          tunnel: [w43] -> w29 mode=indexing
          tunnel: [w42] -> w28 mode=indexing
          i -> [w54]
          stop <- w53 stop-if-true
          n19 = stacked-sequence {
            tunnel: w49 -> [_ w66 _ w79 _ w92 _]
            tunnel: [_ _ _ _ _ _ w147] -> w48
            tunnel: [_ _ _ _ _ _ w148] -> w47
            tunnel: [_ _ _ _ _ _ w146] -> w46
            tunnel: [_ _ _ _ _ _ w145] -> w45
            tunnel: [_ _ _ _ _ _ w144] -> w44
            tunnel: [_ _ _ _ _ _ w143] -> w43
            frame #0 {
              w56 = 0.0
              # "CLNA Set"
              n20 = local read "Bias_LO_equip"() -> (w65:T1)
              n21 = local read "CLNA_SET"() -> (w57:T4)
              n22 = Bundle By Name(cluster=w57, "CLNA State"=1, "SET POL0 LNA1 STAGE1 DRAIN V"=w56, "SET POL0 LNA1 STAGE1 DRAIN C"=w56) -> (w62:T4)
              n23 = Unbundle By Name(w65) -> ("Slave Node in"=w60:cluster{"Address":i16, "Serial Number":i8[]}, "ObjHandle out"=w64:u32, "Cartridge band"=w63:u32, "POL"=w59:u32, "sb"=w58:u32)
              n24 = call "WCA_SET_CLNA.vi"("Cartridge Band"=w63, "Slave Node in"=w60, "ObjHandle in"=w64, "POL"=w59, "sb"=w58, "CLNA_SET"=w62) -> ()  [unwired: 8 in, 2 out]
            }
            frame #1 {
              n25 = Unbundle By Name(w66) -> ("wait (mS)"=w67:dbl)
              n26 = Wait (ms)(milliseconds to wait=w67) -> ()  [unwired: 1 out]
            }
            frame #2 {
              # "CLNA Set"
              n27 = local read "Set VD"() -> (w72:dbl)
              n28 = local read "Set ID"() -> (w73:dbl)
              n29 = local read "Bias_LO_equip"() -> (w78:T1)
              n30 = Bundle By Name(cluster="CLNA_SET", "CLNA State"=1, "SET POL0 LNA1 STAGE1 DRAIN V"=w72, "SET POL0 LNA1 STAGE1 DRAIN C"=w73) -> (w74:T4)
              n31 = Unbundle By Name(w78) -> ("Slave Node in"=w70:cluster{"Address":i16, "Serial Number":i8[]}, "ObjHandle out"=w77:u32, "Cartridge band"=w76:u32, "POL"=w69:u32, "sb"=w68:u32)
              n32 = call "WCA_SET_CLNA.vi"("Cartridge Band"=w76, "Slave Node in"=w70, "ObjHandle in"=w77, "POL"=w69, "sb"=w68, "CLNA_SET"=w74) -> ()  [unwired: 8 in, 2 out]
            }
            frame #3 {
              n33 = Unbundle By Name(w79) -> ("wait (mS)"=w80:dbl)
              n34 = Wait (ms)(milliseconds to wait=w80) -> ()  [unwired: 1 out]
            }
            frame #4 {
              # "CLNA GET"
              n35 = local read "Bias_LO_equip"() -> (w85:T1)
              n36 = Unbundle By Name(w85) -> ("Slave Node in"=w86:cluster{"Address":i16, "Serial Number":i8[]}, "ObjHandle out"=w91:u32, "Cartridge band"=w90:u32, "POL"=w89:u32, "sb"=w88:u32, "WCA_avg"=w87:i32)
              n37 = call "WCA_GET_CLNA.vi"("Cartridge Band"=w90, "Slave Node in"=w86, "ObjHandle in"=w91, "POL"=w89, "sb"=w88, "avg"=w87) -> ("CLNA_monitor"=w84:T7)  [unwired: 7 in, 2 out]
              n38 = Unbundle By Name(w84) -> ("Pol0 LNA1 S1 Drain V [V]"=w83:sgl, "Pol0 LNA1 S1 Drain C [mA]"=w82:sgl, "Pol0 LNA1 S1 Gate V [V]"=w81:sgl)
              n39 = local write "Get ID"(w82) -> ()
              n40 = local write "Get VD"(w83) -> ()
              n41 = local write "Get VG"(w81) -> ()
            }
            frame #5 {
              n42 = Unbundle By Name(w92) -> ("HOT/COLD"=w93:u16)
              n43 = case shown="1" w93 {
                tunnel: w92 -> [w99 w120]
                frame 0, Default {
                  # "HOT/COLDが液体窒素の場合"
                  n44 = local read "Control"() -> (w96:T2)
                  n45 = Unbundle By Name(w96) -> ("mortor設定"=w98:T5, "GPIB_PM"=w94:string)
                  n46 = Index Array(array=w98, index=0) -> (element=w95:T6)
                  n47 = stacked-sequence {
                    tunnel: w99 -> [_ w103 w108 _ w112 w117]
                    tunnel: w95 -> [w101 _ _ w110 _ _]
                    tunnel: w94 -> [_ _ w104 _ _ w113]
                    frame #0 {
                      # "Cold＝＞HOT"
                      n48 = call "__move_motor2.vi"("Moving distance"=50.0, "motor setup"=w101) -> ()  [unwired: 2 in, 2 out]
                    }
                    frame #1 {
                      n49 = Unbundle By Name(w103) -> ("wait (mS)"=w102:dbl)
                      n50 = Wait (ms)(milliseconds to wait=w102) -> ()  [unwired: 1 out]
                    }
                    frame #2 {
                      n51 = Unbundle By Name(w108) -> ("frq(GHz)"=w106:dbl, "P.M.aveg"=w107:i32)
                      n52 = call "__READ_PM_1ch_E4419A_aveg.VI"("aveg"=w107, "frq(GHz)"=w106, "GPIB"=w104) -> ("chA"=w105:dbl)  [unwired: 4 in]
                      n53 = local write "Phot"(w105) -> ()
                    }
                    frame #3 {
                      # "Coldにする"
                      n54 = call "__move_motor2.vi"("Moving distance"=-50, "motor setup"=w110) -> ()  [unwired: 2 in, 2 out]
                    }
                    frame #4 {
                      n55 = Unbundle By Name(w112) -> ("wait (mS)"=w111:dbl)
                      n56 = Wait (ms)(milliseconds to wait=w111) -> ()  [unwired: 1 out]
                    }
                    frame #5 {
                      n57 = Unbundle By Name(w117) -> ("frq(GHz)"=w115:dbl, "P.M.aveg"=w116:i32)
                      n58 = call "__READ_PM_1ch_E4419A_aveg.VI"("aveg"=w116, "frq(GHz)"=w115, "GPIB"=w113) -> ("chA"=w114:dbl)  [unwired: 4 in]
                      n59 = local write "Pcold"(w114) -> ()
                    }
                  }
                }
                frame 1 {
                  # "SISBiasのとき"
                  n60 = local read "Control"() -> (w119:T2)
                  n61 = Unbundle By Name(w119) -> ("GPIB_PM"=w118:string)
                  n62 = stacked-sequence {
                    tunnel: w120 -> [w123 w126 w131 w134 w137 w142]
                    tunnel: w118 -> [_ _ w127 _ _ w138]
                    frame #0 {
                      w124 = 0
                      n63 = local read "Bias_LO_equip"() -> (w121:T1)
                      n64 = Unbundle By Name(w123) -> ("SIS hotV"=w122:dbl)
                      n65 = call "__SISbias_Set.vi"("SIS　Mode"=w124, "Offset"=w124, "Set_V"=w122, "Bias_LO_equip"=w121) -> ()  [unwired: 7 in, 1 out]
                    }
                    frame #1 {
                      n66 = Unbundle By Name(w126) -> ("wait (mS)"=w125:dbl)
                      n67 = Wait (ms)(milliseconds to wait=w125) -> ()  [unwired: 1 out]
                    }
                    frame #2 {
                      n68 = Unbundle By Name(w131) -> ("frq(GHz)"=w129:dbl, "P.M.aveg"=w130:i32)
                      n69 = call "__READ_PM_1ch_E4419A_aveg.VI"("aveg"=w130, "frq(GHz)"=w129, "GPIB"=w127) -> ("chA"=w128:dbl)  [unwired: 4 in]
                      n70 = local write "Phot"(w128) -> ()
                    }
                    frame #3 {
                      w135 = 0
                      n71 = local read "Bias_LO_equip"() -> (w132:T1)
                      n72 = Unbundle By Name(w134) -> ("SIS coldV"=w133:dbl)
                      n73 = call "__SISbias_Set.vi"("SIS　Mode"=w135, "Offset"=w135, "Set_V"=w133, "Bias_LO_equip"=w132) -> ()  [unwired: 7 in, 1 out]
                    }
                    frame #4 {
                      n74 = Unbundle By Name(w137) -> ("wait (mS)"=w136:dbl)
                      n75 = Wait (ms)(milliseconds to wait=w136) -> ()  [unwired: 1 out]
                    }
                    frame #5 {
                      n76 = Unbundle By Name(w142) -> ("frq(GHz)"=w140:dbl, "P.M.aveg"=w141:i32)
                      n77 = call "__READ_PM_1ch_E4419A_aveg.VI"("aveg"=w141, "frq(GHz)"=w140, "GPIB"=w138) -> ("chA"=w139:dbl)  [unwired: 4 in]
                      n78 = local write "Pcold"(w139) -> ()
                    }
                  }
                }
              }
            }
            frame #6 {
              n79 = local read "Pcold"() -> (w144:dbl)
              n80 = local read "Get VG"() -> (w146:dbl)
              n81 = local read "Get ID"() -> (w148:dbl)
              n82 = local read "Get VD"() -> (w147:dbl)
              n83 = local read "Phot"() -> (w145:dbl)
              n84 = Subtract(x=w145, y=w144) -> (x-y=w143:dbl)
              n85 = local write "Y_"(w143) -> ()
            }
          }
          n86 = Unbundle By Name(w49) -> ("IDmin"=w52:dbl, "IDmax"=w51:dbl, "IDstep"=w50:dbl)
          n87 = Multiply(x=w50, y=w54) -> (x*y=w55:dbl)
          n88 = Add(x=w52, y=w55) -> (x+y=w42:dbl)
          n89 = Greater Or Equal?(x=w42, y=w51) -> (x >= y?=w53:bool)
          n90 = local write "Set ID"(w42) -> ()
        }
        n91 = Unbundle By Name(w35) -> ("VDmin"=w38:dbl, "VDmax"=w37:dbl, "VDstep"=w36:dbl)
        n92 = Multiply(x=w36, y=w41) -> (x*y=w40:dbl)
        n93 = Add(x=w38, y=w40) -> (x+y=w27:dbl)
        n94 = Greater Or Equal?(x=w27, y=w37) -> (x >= y?=w39:bool)
        n95 = local write "Set VD"(w27) -> ()
        n96 = local write "SET ID"(w28) -> ()
      }
      n97 = local write "SET VD"(w21) -> ()
      n98 = local write "PH"(w24) -> ()
      n99 = local write "VG"(w25) -> ()
      n100 = local write "PC"(w23) -> ()
      n101 = local write "GetVD 2D"(w20) -> ()
      n102 = local write "Y"(w22) -> ()
      n103 = local write "GETID2d"(w19) -> ()
    }
    frame #2 {
      n104 = local read "Y"() -> (w157:dbl[][])
      n105 = Array Size(array=w157) -> (size(s)=w154:i32[])
      n106 = local read "VG"() -> (w169:dbl[][])
      n107 = Index Array(array=w154, index=1) -> (element=w152:i32)
      n108 = Index Array(array=w154, index=0) -> (element=w153:i32)
      n109 = Decrement(x=w153) -> (x-1=w151:i32)
      n110 = Decrement(x=w152) -> (x-1=w150:i32)
      n111 = local read "PC"() -> (w165:dbl[][])
      n112 = Multiply(x=w151, y=w150) -> (x*y=w149:i32)
      n113 = Reshape Array(w157, w149) -> (w159:dbl[])
      n114 = Reshape Array(w169, w149) -> (w162:dbl[])
      n115 = local read "PH"() -> (w168:dbl[][])
      n116 = Reshape Array(w165, w149) -> (w160:dbl[])
      n117 = Reshape Array(w168, w149) -> (w161:dbl[])
      n118 = local read "GetVD 2D"() -> (w167:dbl[][])
      n119 = Reshape Array(w167, w149) -> (w164:dbl[])
      n120 = local read "GETID2d"() -> (w166:dbl[][])
      n121 = Reshape Array(w166, w149) -> (w163:dbl[])
      n122 = Build Array(w164, w163, w162, w161, w160, w159) -> (w158:dbl[][])
      n123 = local write "AllDATA"(w158) -> ()
    }
    frame #3 {
      n124 = local read "CLNAsweep"() -> (w188:T3)
      n125 = local read "Control"() -> (w172:T2)
      n126 = Unbundle By Name(w188) -> ("VDmin"=w197:dbl, "VDstep"=w196:dbl, "IDmin"=w195:dbl, "IDstep"=w194:dbl)
      n127 = Unbundle By Name(w172) -> ("DATAパス"=w171:path)
      n128 = Unbundle By Name(w188) -> ("file_name"=w222:string)
      n129 = Equal?(x=w171, y=path "") -> (x = y?=w223:bool)
      n130 = Format Into String(format string="matrix using (%.3f+$1*%.3f):(%.3f+$2*%.3f):3", w195, w194, w197, w196) -> (resulting string=w182:string)  [unwired: 2 in, 1 out]
      n131 = String Length(string=w222) -> (length=w228:i32)
      n132 = Equal?(x=w228, y=0) -> (x = y?=w224:bool)
      n133 = Or(x=w224, y=w223) -> (x .or. y?=w225:bool)
      n134 = case shown="참" w225 {
        tunnel: w222 -> [w368 _]
        tunnel: [w370 w376] -> w206
        tunnel: [FALSE w377] -> _
        tunnel: w171 -> [w369 _]
        tunnel: [w369 w374] -> w185
        tunnel: [w368 w373] -> w184
        frame False {
          n135 = Build Path(base path=w369, name or relative path=w368) -> (appended path=w371:path)
          n136 = Open/Create/Replace File(file path (use dialog)=w371) -> (refnum out=w370:refnum<file>)  [unwired: 5 in, 2 out]
        }
        frame True {
          n137 = Open/Create/Replace File(operation (0:open)=5) -> (refnum out=w376:refnum<file>, cancelled=w377:bool)  [unwired: 5 in, 1 out]
          n138 = Refnum to Path(1:w376) -> (0:w375:path)
          n139 = Strip Path(path=w375) -> (stripped path=w374:path, name=w373:string)
        }
      }
      n140 = local read "Control"() -> (w173:T2)
      n141 = Concatenate Strings("Trx_", w184) -> (w181:string)
      n142 = Concatenate Strings("VG_", w184) -> (w192:string)
      n143 = Concatenate Strings("PH_", w184) -> (w191:string)
      n144 = Concatenate Strings("VD_", w184) -> (w210:string)
      n145 = Concatenate Strings("ID_", w184) -> (w193:string)
      n146 = Concatenate Strings("Y_", w184) -> (w190:string)
      n147 = Concatenate Strings("ALL_", w184) -> (w198:string)
      n148 = Build Path(base path=w185, name or relative path=w181) -> (appended path=w183:path)
      n149 = Build Path(base path=w185, name or relative path=w192) -> (appended path=w215:path)
      n150 = Build Path(base path=w185, name or relative path=w210) -> (appended path=w221:path)
      n151 = Build Path(base path=w185, name or relative path=w193) -> (appended path=w218:path)
      n152 = Build Path(base path=w185, name or relative path=w191) -> (appended path=w216:path)
      n153 = Build Path(base path=w185, name or relative path=w190) -> (appended path=w214:path)
      n154 = Build Path(base path=w185, name or relative path=w198) -> (appended path=w212:path)
      n155 = local read "GetVD 2D"() -> (w220:dbl[][])
      n156 = local read "GETID2d"() -> (w219:dbl[][])
      n157 = local read "AllDATA"() -> (w213:dbl[][])
      n158 = local read "PH"() -> (w180:dbl[][])
      n159 = local read "VG"() -> (w217:dbl[][])
      n160 = local read "Y"() -> (w189:dbl[][])
      n161 = Unbundle By Name(w173) -> ("Th"=w178:dbl, "Tc"=w177:dbl)
      n162 = local read "PC"() -> (w176:dbl[][])
      n163 = call-poly <vilib>:"Write To Spreadsheet File.vi"("2D data"=w217, "file path (dialog if empty)"=w215) -> ()  [unwired: 6 in, 1 out]
      n164 = call-poly <vilib>:"Write To Spreadsheet File.vi"("2D data"=w220, "file path (dialog if empty)"=w221) -> ()  [unwired: 6 in, 1 out]
      n165 = call-poly <vilib>:"Write To Spreadsheet File.vi"("2D data"=w219, "file path (dialog if empty)"=w218) -> ()  [unwired: 6 in, 1 out]
      n166 = call-poly <vilib>:"Write To Spreadsheet File.vi"("2D data"=w180, "file path (dialog if empty)"=w216) -> ()  [unwired: 6 in, 1 out]
      n167 = call-poly <vilib>:"Write To Spreadsheet File.vi"("2D data"=w189, "file path (dialog if empty)"=w214) -> ()  [unwired: 6 in, 1 out]
      n168 = call-poly <vilib>:"Write To Spreadsheet File.vi"("2D data"=w213, "file path (dialog if empty)"=w212) -> ()  [unwired: 6 in, 1 out]
      n169 = call "ダイナミックデータへ変換"("2D Array"=w180) -> ("Dynamic Data Type"=w179:dynamicdata)  [unwired: 3 in]
      n170 = call "ダイナミックデータへ変換2"("2D Array"=w176) -> ("Dynamic Data Type"=w175:dynamicdata)  [unwired: 3 in]
      n171 = xnode "フォーミュラ"("Ph"=w179, "Pc"=w175, "th"=w178, "tc"=w177) -> ("結果"=w174:dynamicdata)  [unwired: 1 in, 1 out]
      n172 = call "ダイナミックデータから変換"("Dynamic Data Type"=w174) -> ("Array"=w187:dbl[][])  [unwired: 3 in]
      n173 = Format Into String(format string="set title    \"VD(V)\"\nsplot  \\'%s\\' %s  with lines\\n\npause -1 \\n\nset title    \"ID(mA)\"\nsplot  \\'%s\\' %s  with lines\\n\npause -1 \\n\nset title    \"VG(V)\"\nsplot  \\'%s\\' %s  with lines\\n\npause -1 \\n\nset title    \"PH(dBm)\"\nsplot  \\'%s\\' %s  with lines\\n\npause -1 \\n\nset title    \"Y(dB)\"\nsplot  \\'%s\\' %s  with lines\\n\npause -1 \\n\nset zrange [100:600]\nset title    \"Trx(k)\"\nsplot  \\'%s\\' %s  with lines\\n\npause -1 \\n\n", w210, w182, w193, w182, w192, w182, w191, w182, w190, w182, w181, w182) -> (resulting string=w208:string)  [unwired: 2 in, 1 out]
      n174 = Concatenate Strings("reset \nset contour base\nunset surface\nset key off\nset xlabel  \"ID(mA)\"  \n set ylabel  \"VD(V)\"\nset pm3d at b\n", w208) -> (w207:string)
      n175 = call-poly <vilib>:"Write To Spreadsheet File.vi"("2D data"=w187, "file path (dialog if empty)"=w183) -> ()  [unwired: 6 in, 1 out]
      n176 = Write to Text File(file (use dialog)=w206, text=w207) -> (refnum out=w170:refnum<file>)  [unwired: 2 in, 2 out]
      n177 = Close File(refnum=w170) -> ()  [unwired: 1 in, 2 out]
    }
    frame #4 {
      n178 = local read "Link済み"() -> (w379:bool)
      n179 = case shown="거짓" w379 {
        frame False {
          n180 = local read "Bias_LO_equip"() -> (w382:T1)
          n181 = Unbundle By Name(w382) -> ("ObjHandle out"=w381:u32)
          n182 = call "WCA_CAN_close.vi"("ObjHandle in"=w381) -> ()  [unwired: 14 in, 1 out]
          n183 = local write "Link済み"(FALSE) -> ()
        }
        frame True {
        }
      }
    }
  }
